vi "Read Max Qorf DVR.vi"(8 "error in (no error)":errorcluster, 11 "O3 Cal State in":refnum<class "O3 Cal State.lvclass">) -> (0 "error out":errorcluster, 2 "Max Qorf DVR":refnum<data-value>, 3 "O3 Cal State out":refnum<class "O3 Cal State.lvclass">)   [LabVIEW 2012, in "O3 Cal State.lvclass"]
uses:
  O3 Cal State.lvclass
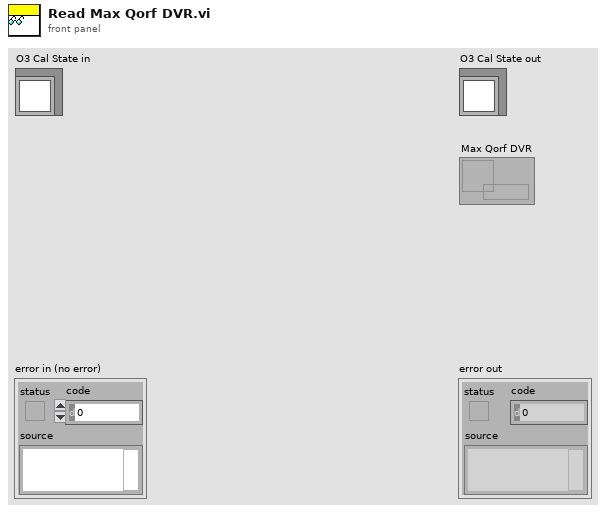
[diagram p1: front panel]
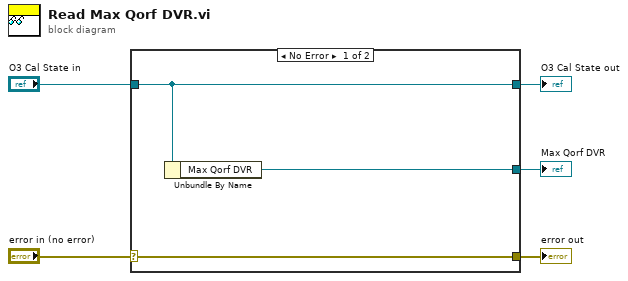
[diagram p0: block diagram]
diagram:
  n1 = case shown="No Error" "error in (no error)" {
    selector: "error in (no error)" -> [w8 w9]
    tunnel: [w8 w9] -> w4
    tunnel: [w7 w10] -> w2
    tunnel: "O3 Cal State in" -> [w7 w10]
    tunnel: [w6 _] -> w1
    frame No Error {
      n2 = Unbundle By Name(w7) -> ("Max Qorf DVR"=w6:refnum<data-value>)
    }
    frame Error {
    }
  }
  "error out" <- w4
  "O3 Cal State out" <- w2
  "Max Qorf DVR" <- w1
